vi "PGPASS.Format Connection String.vi"(8 "error in":errorcluster, 11 "Connection Information":T1) -> (0 "error out":errorcluster, 3 "connection string":string)   [LabVIEW 2019, in "PGPASS.lvlib"]
uses:
  PGPASS.lvlib
  PGPASS.Connection Information.ctl
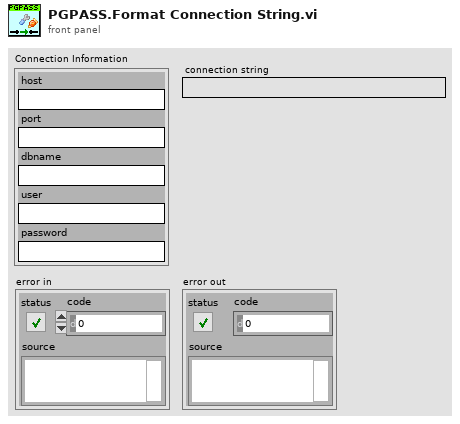
[diagram p1: front panel]
types:
  T1 = typedef "PGPASS.lvlib/PGPASS.Connection Information.ctl" = cluster{"host":string, "port":string, "dbname":string, "user":string, "password":string}
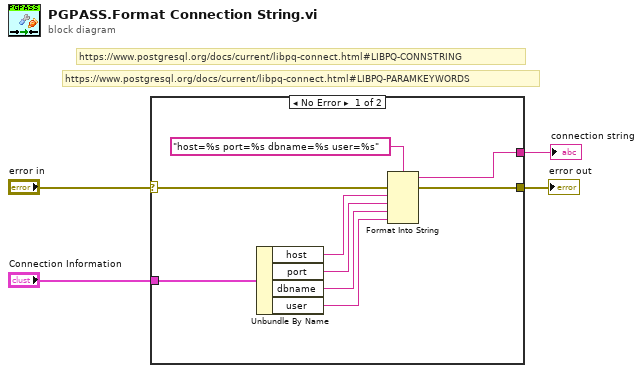
[diagram p0: block diagram]
diagram:
  # "https://www.postgresql.org/docs/current/libpq-connect.html#LIBPQ-PARAMKEYWORDS"
  # "https://www.postgresql.org/docs/current/libpq-connect.html#LIBPQ-CONNSTRING"
  n1 = case shown="No Error" "error in" {
    selector: "error in" -> [w5 w14]
    tunnel: "Connection Information" -> [w12 _]
    tunnel: [w7 _] -> w3
    tunnel: [w6 w14] -> w2
    frame No Error {
      n2 = Unbundle By Name(w12) -> ("host"=w11:string, "port"=w10:string, "dbname"=w9:string, "user"=w8:string)
      n3 = Format Into String(format string="host=%s port=%s dbname=%s user=%s", error in=w5, w11, w10, w9, w8) -> (resulting string=w7:string, error out=w6:errorcluster)  [unwired: 1 in]
    }
    frame Error {
    }
  }
  "connection string" <- w3
  "error out" <- w2
